vi "Regular Timer Kernel.vi"(8 "error in":errorcluster, 9 "Timer Data In":T1, 10 "Time Target":dbl, 11 "Enum":T2) -> (0 "error out":errorcluster, 2 "Timer Data Out":T1, 3 "Status":cluster{"Running":bool, "Done":bool})   [LabVIEW 2014]
uses:
  Control Timer.ctl
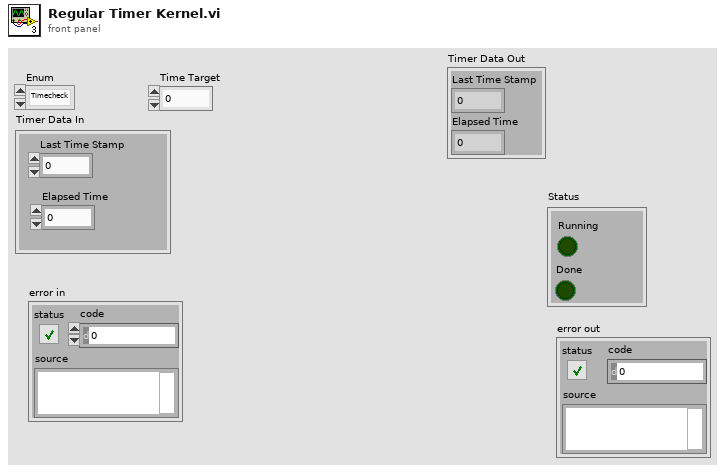
[diagram p1: front panel]
types:
  T1 = cluster{"Last Time Stamp":dbl, "Elapsed Time":dbl}
  T2 = typedef "Control Timer.ctl" = enum16{"Timecheck", "Reset"}
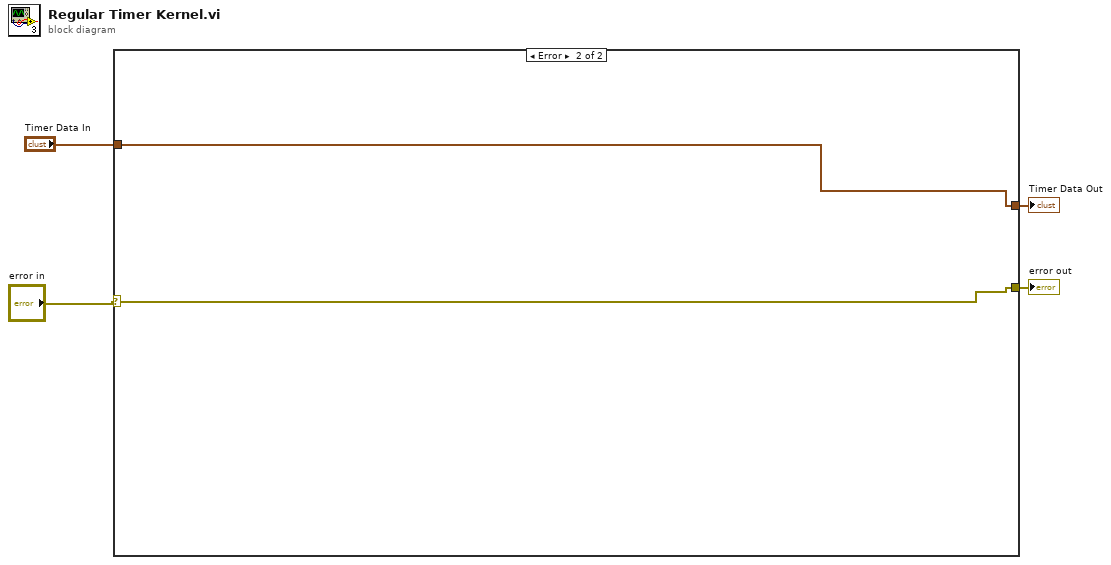
[diagram p0: block diagram]
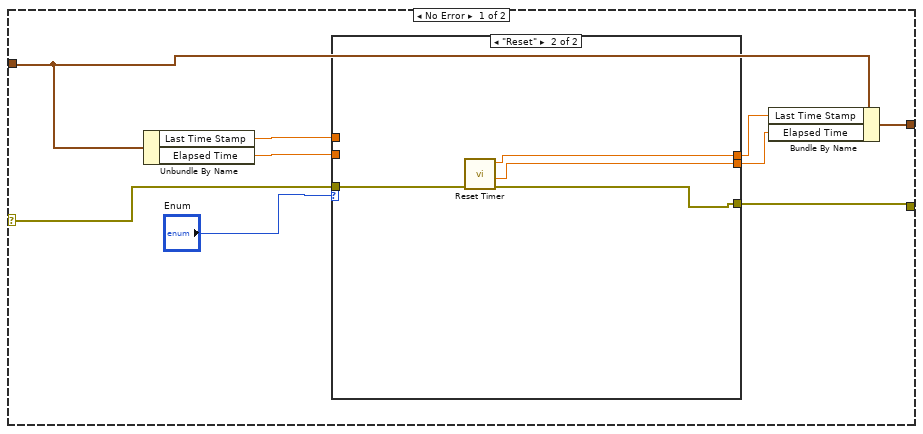
[diagram p2: hidden frame]
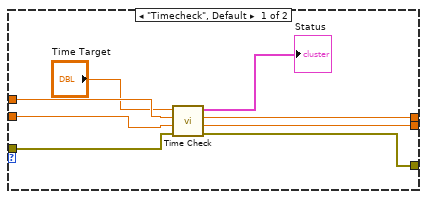
[diagram p3: hidden frame]
diagram:
  n1 = case shown="Error" "error in" {
    selector: "error in" -> [w10 w27]
    tunnel: [w9 w27] -> w3
    tunnel: [w6 w26] -> w2
    tunnel: "Timer Data In" -> [w5 w26]
    frame No Error {
      n2 = Unbundle By Name(w5) -> ("Last Time Stamp"=w12:dbl, "Elapsed Time"=w11:dbl)
      n3 = case shown="\"Reset\"" "Enum" {
        tunnel: w12 -> [w21 _]
        tunnel: w11 -> [w20 _]
        tunnel: w10 -> [w19 w25]
        tunnel: [w18 w24] -> w9
        tunnel: [w17 w22] -> w8
        tunnel: [w16 w23] -> w7
        frame "Timecheck", Default {
          n4 = call "Time Check.vi"("error in"=w19, "Elapsed Time"=w20, "Last Time Stamp"=w21, "Time Target"="Time Target") -> ("error out"=w18:errorcluster, "New Elapsed Time"=w16:dbl, "New Time Stamp"=w17:dbl, "Status"=→"Status":cluster{"Running":bool, "Done":bool})  [unwired: 3 in]
        }
        frame "Reset" {
          n5 = call "Reset Timer.vi"("error in"=w25) -> ("error out"=w24:errorcluster, "New Elapsed Time"=w23:dbl, "New Time Stamp"=w22:dbl)  [unwired: 8 in]
        }
      }
      n6 = Bundle By Name(cluster=w5, "Last Time Stamp"=w8, "Elapsed Time"=w7) -> (w6:T1)
    }
    frame Error {
    }
  }
  "error out" <- w3
  "Timer Data Out" <- w2
